vi "Write_CmdDiagnostic.vi"(8 "error in (no error)":errorcluster, 10 "Command":enum16{"# ?", "TRG", "RST", "GTM", "GVM"}(ring), 11 "Multiplexer_Opmux in":refnum<class "Multiplexer_Opmux.lvclass">) -> (0 "error out":errorcluster, 3 "Multiplexer_Opmux out":refnum<class "Multiplexer_Opmux.lvclass">)   [LabVIEW 2014, in "Multiplexer_Opmux.lvclass"]
uses:
  Multiplexer_Opmux.lvclass
  Multiplexer_Opmux.lvclass/Multiplexer_Opmux.ctl
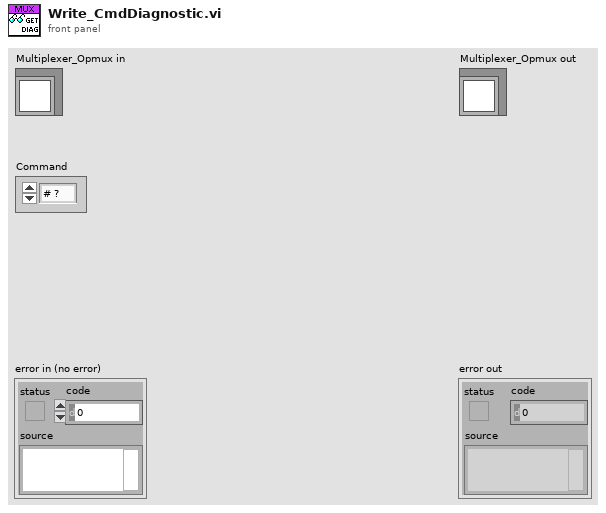
[diagram p1: front panel]
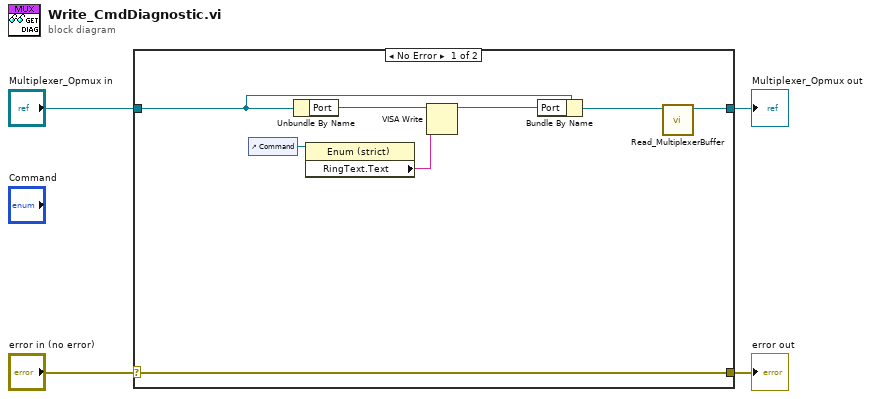
[diagram p0: block diagram]
diagram:
  n1 = case shown="No Error" "error in (no error)" {
    selector: "error in (no error)" -> [w12 w14]
    tunnel: [w12 w14] -> w3
    tunnel: [w8 w13] -> w1
    tunnel: "Multiplexer_Opmux in" -> [w6 w13]
    frame No Error {
      n2 = control-ref of="Command"() -> (w11:refnum<vi>)
      n3 = Unbundle By Name(w6) -> ("Port"=w9:refnum<visa-resource-name>)
      n4 = property class="Enum (strict)"(reference=w11) -> ("RingText.Text"=w10:string)  [unwired: 1 in, 2 out]
      n5 = VISA Write(VISA resource name=w9, write buffer=w10) -> (VISA resource name out=w5:refnum<visa-resource-name>)  [unwired: 1 in, 2 out]
      n6 = Bundle By Name(cluster=w6, "Port"=w5) -> (w7:refnum<class "Multiplexer_Opmux.lvclass">)
      n7 = call-dynamic "Read_MultiplexerBuffer.vi"("Multiplexer_Opmux in"=w7) -> ("Multiplexer_Opmux out"=w8:refnum<class "Multiplexer_Opmux.lvclass">)  [unwired: 8 in, 2 out]
    }
    frame Error {
    }
  }
  "error out" <- w3
  "Multiplexer_Opmux out" <- w1
